vi "State Machine.vi"() -> ()   [LabVIEW 2015]
uses:
  State Enum.ctl
panel:
  in  "Menu":T1
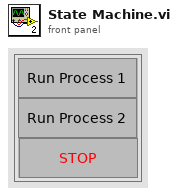
[diagram p1: front panel]
types:
  T1 = cluster{"Process 1":bool, "Process 2":bool, "stop":bool}
  T2 = typedef "State Enum.ctl" = enum32{"Idle", "Process 1", "Process 2", "Stop"}
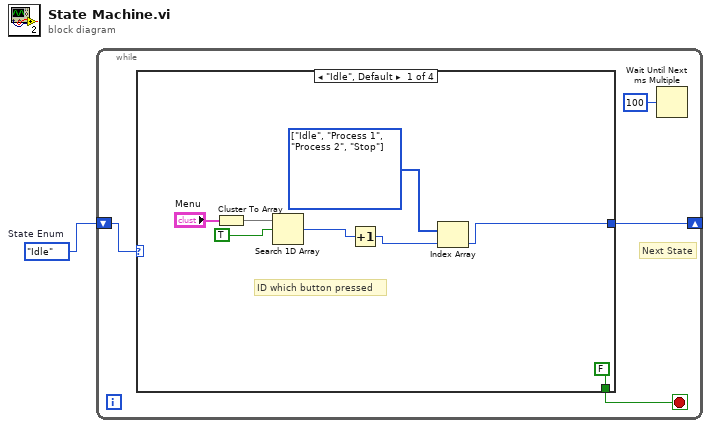
[diagram p0: block diagram]
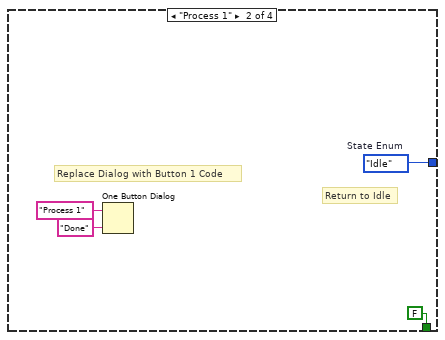
[diagram p2: hidden frame]
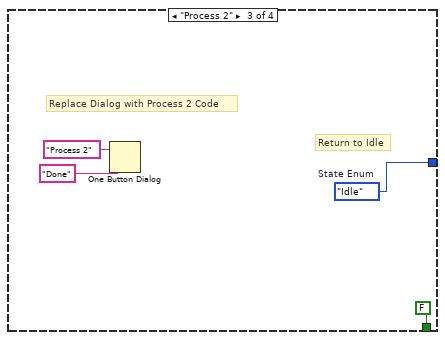
[diagram p3: hidden frame]
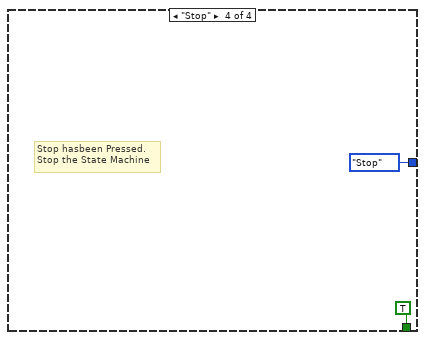
[diagram p4: hidden frame]
diagram:
  w1 = State_Enum."Idle"  # State Enum
  n1 = while {
    shift-right: [w3] -> _
    shift-left: w1 -> [w4]
    stop <- w5 stop-if-true
    # "Next State"
    n2 = case shown="\"Idle\", Default" w4 {
      tunnel: [FALSE FALSE FALSE TRUE] -> w5
      tunnel: [w9 w16 w19 State_Enum."Stop" ("State Enum")] -> w3
      frame "Idle", Default {
        w10 = T2[] [enum."Idle", enum."Process 1", enum."Process 2", enum."Stop"] items=["Idle", "Process 1", "Process 2", "Stop"]
        # "ID which button pressed"
        n3 = Cluster To Array(cluster="Menu") -> (array=w12:bool[])
        n4 = Search 1D Array(1D array=w12, element=TRUE) -> (index of element=w7:i32)  [unwired: 1 in]
        n5 = Increment(x=w7) -> (x+1=w6:i32)
        n6 = Index Array(array=w10, index=w6) -> (element=w9:T2)
      }
      frame "Process 1" {
        w16 = State_Enum."Idle"  # State Enum
        # "Return to Idle"
        # "Replace Dialog with Button 1 Code"
        n7 = One Button Dialog(message="Process 1", button name ("OK")="Done") -> ()  [unwired: 1 out]
      }
      frame "Process 2" {
        w19 = State_Enum."Idle"  # State Enum
        # "Return to Idle"
        # "Replace Dialog with Process 2 Code"
        n8 = One Button Dialog(message="Process 2", button name ("OK")="Done") -> ()  [unwired: 1 out]
      }
      frame "Stop" {
        # "Stop hasbeen Pressed.\nStop the State Machine"
      }
    }
    n9 = Wait Until Next ms Multiple(millisecond multiple=u32 100) -> ()  [unwired: 1 out]
  }
